vi "Read stop.vi"(8 "error in (no error)":errorcluster, 11 "Master CR in":refnum<class "WebSocket Client CR.lvclass">) -> (0 "error out":errorcluster, 2 "Stop":bool, 3 "Master CR out":refnum<class "WebSocket Client CR.lvclass">)   [LabVIEW 2021, in "WebSockets.lvlib" / "WebSocket Client CR.lvclass"]
uses:
  WebSocket Client CR.lvclass
  WebSocket Client CR.lvclass/WebSocket Client CR.ctl
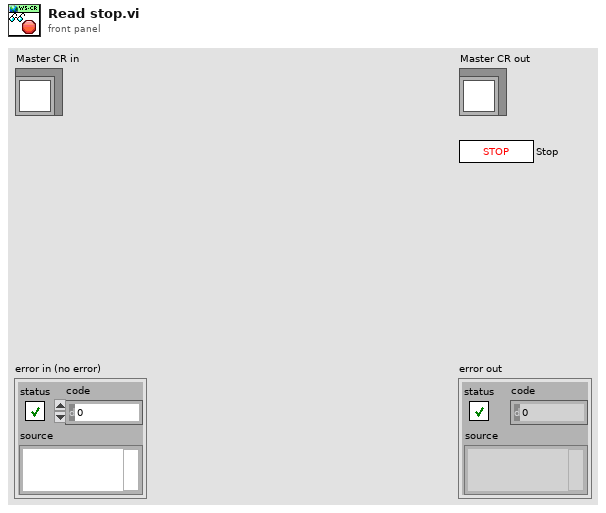
[diagram p1: front panel]
types:
  T1 = typedef "WebSockets.lvlib/WebSocket Client CR.lvclass/Master CR state.ctl" = cluster{"state":T2, "enable":bool, "write enable":bool, "connect":bool, "errors":i32, "Run":bool, "Write":bool, "Stop":bool}
  T2 = typedef "WebSockets.lvlib/WebSocket Client CR.lvclass/CR_Core_State.ctl" = enum8{"initialization", "redefine", "standby", "ping", "connect", "wait to reconnect", "wait to reset timeout", "configure", "requests", "close connection", "stop"}
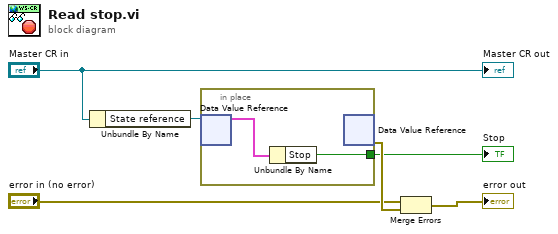
[diagram p0: block diagram]
diagram:
  n1 = Unbundle By Name("Master CR in") -> ("State reference"=w6:refnum<data-value>)
  n2 = in-place {
    in-place-border: [w8] -> w3
    n3 = in-place-dvr #1(w6) -> (w7:T1)  [unwired: 1 out]
    n4 = Unbundle By Name(w7) -> ("Stop"=w8:bool)
    n5 = in-place-dvr #1() -> (w5:errorcluster)  [unwired: 1 in, 1 out]
  }
  "Stop" <- w3
  n6 = Merge Errors("error in (no error)", w5) -> (→"error out":errorcluster)
  "Master CR out" <- "Master CR in"
